vi "provide_OME_data.vi"(6 "image ID":string, 8 "error in (no error)":errorcluster, 9 "structuredAttribute string in":string, 10 "OME element in":refnum<class "XMLElement.lvclass">, 11 "YK090623DAQmxAnalogDetector in":refnum<class "DetectorYK090623DAQmxAnalog.lvclass">) -> (0 "error out":errorcluster, 1 "structuredAttribute string out":string, 2 "OME element out":refnum<class "XMLElement.lvclass">, 3 "YK090623DAQmxAnalogDetector out":refnum<class "DetectorYK090623DAQmxAnalog.lvclass">)   [LabVIEW 2010, in "DetectorYK090623DAQmxAnalog.lvclass"]
uses:
  DetectorYK090623DAQmxAnalog.lvclass
  common/classes/XMLElement/XMLElement/XMLElement.lvclass
  GenericDetector/GenericDetector/GenericDetector.lvclass
  DetectorYK090623DAQmxAnalog.lvclass/DetectorYK090623DAQmxAnalog.ctl
  common/classes/ErrorController/ErrorController/class_data.vi
  Instrument/GenericInstrument/GenericInstrument/GenericInstrument.lvclass
  common/classes/ErrorController/ErrorController/ErrorController.lvclass
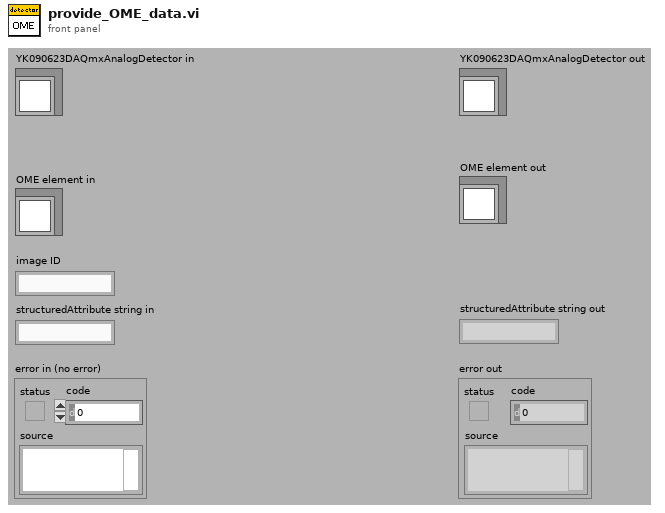
[diagram p1: front panel]
types:
  T1 = typedef "GenericDetector.lvclass/type_enum.ctl" = enum16{"CCD", "IntensifiedCCD", "AnalogVideo", "PMT", "Photodiode", "Spectoscropy", "LifetimeImaging", "CorrelationSpectroscopy", "FTIR", "EM-CCD", "APD", "CMOS", "Unknown"}
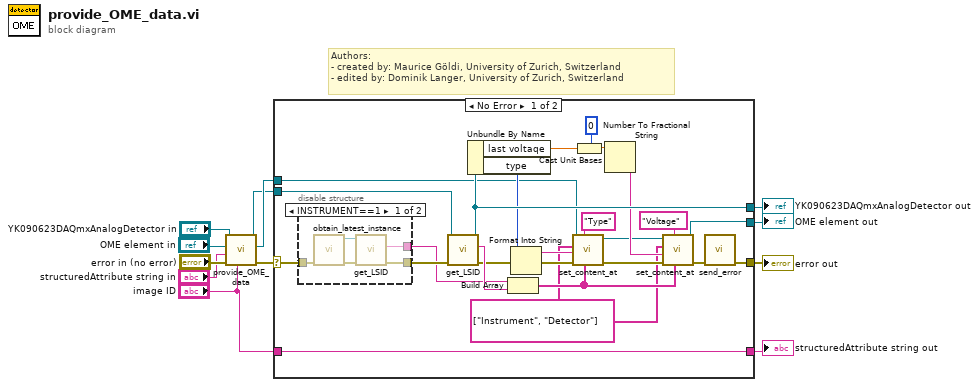
[diagram p0: block diagram]
diagram:
  # "Authors: \n- created by: Maurice Göldi, University of Zurich, Switzerland\n- edited by: Dominik Langer, University of Zurich, Switzerland"
  n1 = call-parent "provide_OME_data.vi"("image ID"="image ID", "error in (no error)"="error in (no error)", "structuredAttribute string in"="structuredAttribute string in", "OME element in"="OME element in", "GenericPlugin in"="YK090623DAQmxAnalogDetector in") -> ("error out"=w9:errorcluster, "OME element out"=w8:refnum<class "XMLElement.lvclass">, "GenericPlugin out"=w6:refnum<class "DetectorYK090623DAQmxAnalog.lvclass">)  [unwired: 3 in, 1 out]
  n2 = case shown="No Error" w9 {
    selector: w9 -> [w31 w47]
    tunnel: [w26 w47] -> w12
    tunnel: [w33 w46] -> w11
    tunnel: w6 -> [w34 w46]
    tunnel: w8 -> [w15 w45]
    tunnel: [w28 w45] -> w4
    tunnel: "image ID" -> [w23 w44]
    tunnel: [w23 w44] -> w1
    frame No Error {
      w13 = string[] ["Instrument", "Detector"]
      n3 = disable-structure shown="INSTRUMENT==1" {
        disable-tunnel: w31 -> [w40 w43]
        disable-tunnel: [w39 w43] -> w30
        disable-tunnel: [w38 _] -> w29
        frame condition #0 {
          n4 = call "obtain_latest_instance.vi"("error in (no error)"=w40) -> ("error out"=w41:errorcluster, "microscope"=w42:refnum<class "GenericInstrument.lvclass">)  [unwired: 9 in]
          n5 = call-dynamic "get_LSID.vi"("error in (no error)"=w41, "GenericPlugin in"=w42) -> ("error out"=w39:errorcluster, "LSID (string)"=w38:string)  [unwired: 6 in, 2 out]
        }
        frame condition #1 (active) {
        }
      }
      n6 = call-dynamic "get_LSID.vi"("error in (no error)"=w30, "GenericPlugin in"=w34) -> ("error out"=w19:errorcluster, "LSID (string)"=w32:string, "GenericPlugin out"=w33:refnum<class "DetectorYK090623DAQmxAnalog.lvclass">)  [unwired: 6 in, 1 out]
      n7 = Unbundle By Name(w33) -> ("last voltaqe"=w37:dbl[unit], "type"=w16:T1)
      n8 = Build Array(w29, w32) -> (w17:string[])
      n9 = Format Into String(error in=w19, w16) -> (resulting string=w21:string, error out=w22:errorcluster)  [unwired: 2 in]
      n10 = call "set_content_at.vi"("id chain"=w17, "attribute name"="Type", "error in (no error)"=w22, "content"=w21, "key chain"=w13, "Element in"=w15) -> ("error out"=w18:errorcluster, "Element out"=w14:refnum<class "XMLElement.lvclass">)  [unwired: 4 in]
      n11 = Cast Unit Bases(0:w37, 1:0) -> (2:w36:dbl)
      n12 = Number To Fractional String(number=w36) -> (F-format string=w24:string)  [unwired: 3 in]
      n13 = call "set_content_at.vi"("id chain"=w17, "attribute name"="Voltage", "error in (no error)"=w18, "content"=w24, "key chain"=w13, "Element in"=w14) -> ("error out"=w27:errorcluster, "Element out"=w28:refnum<class "XMLElement.lvclass">)  [unwired: 4 in]
      n14 = call "send_error.vi"("error in (no error)"=w27) -> ("error out"=w26:errorcluster)  [unwired: 10 in]
    }
    frame Error {
    }
  }
  "error out" <- w12
  "YK090623DAQmxAnalogDetector out" <- w11
  "OME element out" <- w4
  "structuredAttribute string out" <- w1
